vi "Test voltage to diameter solution.vi"() -> ()   [LabVIEW 2014, in "DMA.lvclass"]
uses:
  DMA.lvclass
  NOAA Wide/NOAA Wide.lvclass
  DMA.lvclass/DMA.ctl
  Atmospheric/Gas Properties/Gas Properties.lvclass/Gas Properties.ctl
  Particle Class/Particle Properties.lvclass/Particle Properties.ctl
  Accessors/Write Qex.vi
  Accessors/Write Qsh.vi
  Accessors/Read Gas Ref.vi
  Accessors/Read Particle.vi
  Atmospheric/Gas Properties/Accessors/Write P (mb).vi
  Atmospheric/Gas Properties/Accessors/Write T (K).vi
  Particle Class/Accessors/Write D.vi
  <vilib>/Analysis/1siggen.llb/Ramp Pattern by Delta.vi
  Conversion Constants.vi
  Particle Class/Calculate Cc.vi
  Particle Class/Calculate Electric Mobility.vi
  <vilib>/Utility/file.llb/Write To Spreadsheet File (DBL).vi
  Atmospheric/Gas Properties/Gas Properties.lvclass
  Particle Class/Particle Properties.lvclass
  <vilib>/Analysis/NI_AALBase.lvlib
panel:
  out "data  2":cluster{"Ramp Pattern":dbl[], dbl[]}(graph)
  out "appended array":cluster{dbl[], dbl[]}[](array[cluster])
  out "Viscocity":dbl
  in  "Write?":bool
  out "data":cluster{"Ramp Pattern":dbl[], dbl[]}[](graph)
  in  "Qsh":dbl=10.0 format="%#_13g"
  in  "T (K)":dbl=293.15 format="%#_13g"
  in  "P (Pa)":dbl=101000.0 format="%#_13g"
  out "error out":errorcluster
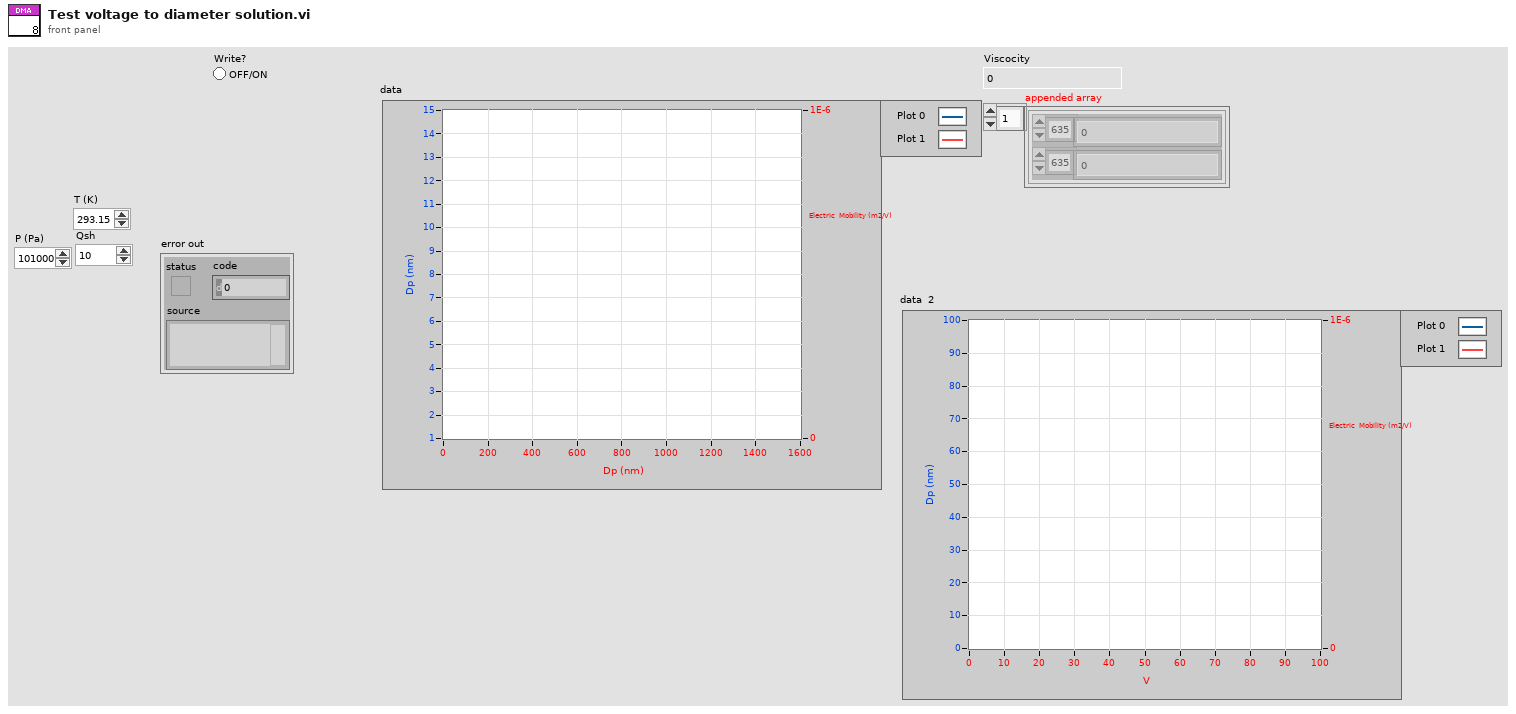
[diagram p1: front panel]
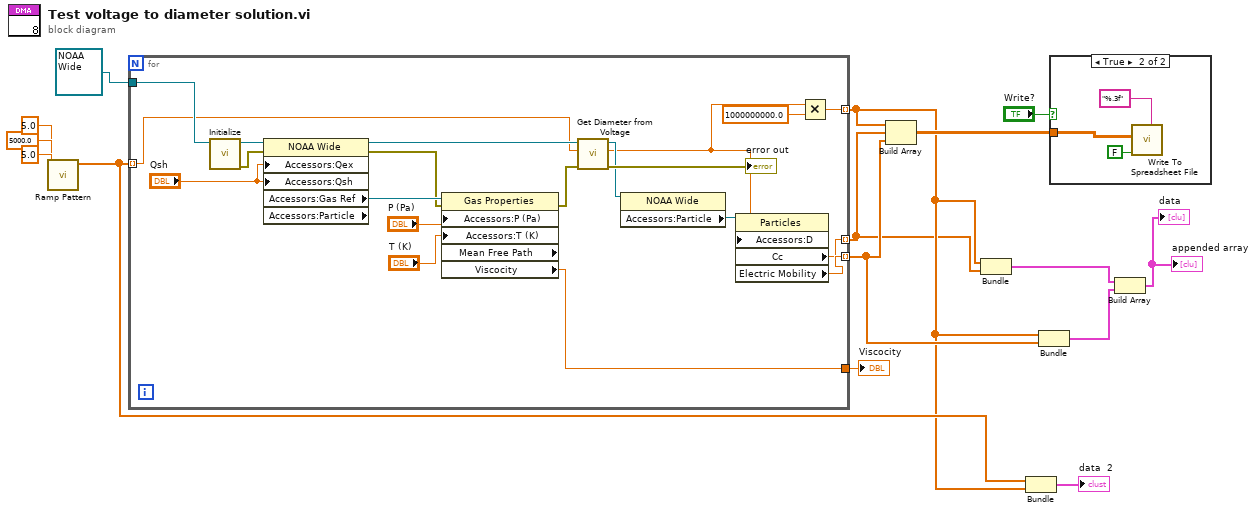
[diagram p0: block diagram]
diagram:
  n1 = call-poly <vilib>:"Ramp Pattern.vi"("start"=5.0, "end"=5000.0, "delta"=5.0) -> ("Ramp Pattern"=w10:dbl[])  [unwired: 6 in, 2 out]
  n2 = for {
    tunnel: [w25] -> w4 mode=indexing
    tunnel: refnum<class "NOAA Wide.lvclass"> refnum ("NOAA Wide") -> [w24]
    tunnel: [w17] -> w3 mode=indexing
    tunnel: [w19] -> w9 mode=indexing
    tunnel: w10 -> [w20] mode=indexing
    tunnel: [w18] -> w5
    n3 = call-dynamic "Initialize.vi"("NOAA Wide in"=w24) -> ("error out"=w30:errorcluster, "NOAA Wide out"=w35:refnum<class "NOAA Wide.lvclass">)  [unwired: 9 in]
    n4 = property class="NOAA Wide" props=["Accessors:Qex", "Accessors:Qsh", "Accessors:Gas Ref", "Accessors:Particle"](reference=w35, error in=w30, "Accessors:Qex"="Qsh", "Accessors:Qsh"="Qsh") -> (reference out=w29:refnum<class "NOAA Wide.lvclass">, error out=w31:errorcluster, "Accessors:Gas Ref"=w34:refnum<data-value>)  [unwired: 1 out]
    n5 = property class="Gas Properties" props=["Accessors:P (Pa)", "Accessors:T (K)", "Mean Free Path", "Viscocity"](reference=w34, error in=w31, "Accessors:P (Pa)"="P (Pa)", "Accessors:T (K)"="T (K)") -> (error out=w28:errorcluster, "Viscocity"=w18:dbl)  [unwired: 2 out]
    n6 = call "Get Diameter from Voltage.vi"("error in"=w28, "Vin"=w20, "DMA in"=w29) -> ("error out"=→"error out":errorcluster, "Dout"=w16:dbl, "DMA out"=w22:refnum<class "NOAA Wide.lvclass">)  [unwired: 6 in]
    n7 = property class="NOAA Wide"(reference=w22) -> ("Accessors:Particle"=w21:refnum<class "Particle Properties.lvclass">)  [unwired: 1 in, 2 out]
    n8 = property class="Particles"(reference=w21, "Accessors:D"=w16) -> ("Cc"=w17:dbl, "Electric Mobility"=w19:dbl)  [unwired: 1 in, 2 out]
    n9 = Multiply(x=w16, y=1000000000.0) -> (x*y=w25:dbl)
  }
  "Viscocity" <- w5
  n10 = Build Array(w4, w3, w9) -> (w14:dbl[][])
  n11 = Bundle(w4, w3) -> (w2:cluster{dbl[], dbl[]})  [unwired: 1 in]
  n12 = Bundle("Ramp Pattern"=w10, w4) -> (→"data  2":cluster{"Ramp Pattern":dbl[], dbl[]})  [unwired: 1 in]
  n13 = Bundle(w4, w9) -> (w8:cluster{dbl[], dbl[]})  [unwired: 1 in]
  n14 = case shown="True" "Write?" {
    tunnel: w14 -> [_ w38]
    frame False {
    }
    frame True {
      n15 = call-poly <vilib>:"Write To Spreadsheet File.vi"("format (%.3f)"="%.3f", "append to file? (new file:F)"=FALSE, "2D data"=w38) -> ()  [unwired: 5 in, 1 out]
    }
  }
  n16 = Build Array(w2, w8) -> (→"data" →"appended array":cluster{dbl[], dbl[]}[])
